vi "一维数组查找最大最小值子VI.vi"(3 "数组 3":dbl[](array[numeric])=[0.0, 0.0, 0.0, 0.0, 0.0, 0.0, 0.0, 7.0, 8.0, 9.0, 0.0, 0.0, 0.0]) -> (0 "最小值":dbl, 1 "最大值":dbl)   [LabVIEW 2013]
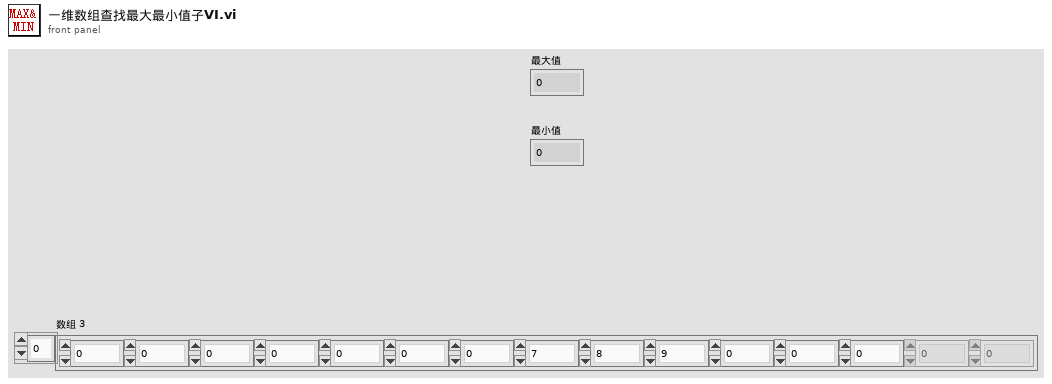
[diagram p1: front panel]
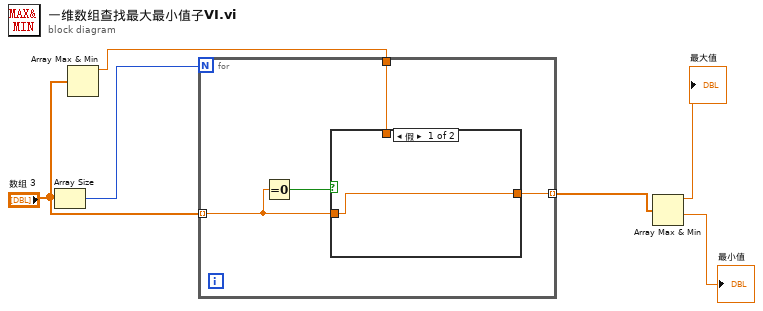
[diagram p0: block diagram]
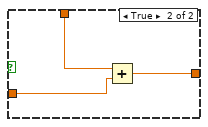
[diagram p2: hidden frame]
diagram:
  n1 = Array Size(array="数组 3") -> (size(s)=w6:i32)
  n2 = Array Max & Min(array="数组 3") -> (max value=w4:dbl)  [unwired: 3 out]
  n3 = for {
    N: w6 -> [_]
    tunnel: "数组 3" -> [w9] mode=indexing
    tunnel: w4 -> [w8]
    tunnel: [w7] -> w3 mode=indexing
    n4 = Equal To 0?(x=w9) -> (x = 0?=w10:bool)
    n5 = case shown="假" w10 {
      tunnel: w9 -> [w11 w14]
      tunnel: w8 -> [_ w13]
      tunnel: [w11 w12] -> w7
      frame False {
      }
      frame True {
        n6 = Add(x=w13, y=w14) -> (x+y=w12:dbl)
      }
    }
  }
  n7 = Array Max & Min(array=w3) -> (max value=→"最大值":dbl, min value=→"最小值":dbl)  [unwired: 2 out]
